vi "Get Selected Controls.vi"(8 "error in (no error)":errorcluster, 10 "List of Properties":string[](array[string]), 11 "Data in":T2) -> (0 "error out":errorcluster, 3 "Selected Ctrls":T1)   [LabVIEW 2020, in "Control Property Tree.lvlib"]
uses:
  Control Property Tree.lvlib
  Module Data--cluster.ctl
  Ctrl Properties Map Data.ctl
  Property array.ctl
  Selected Ctrls - List of Controls.ctl
  Selected Ctrls - List of Properties.ctl
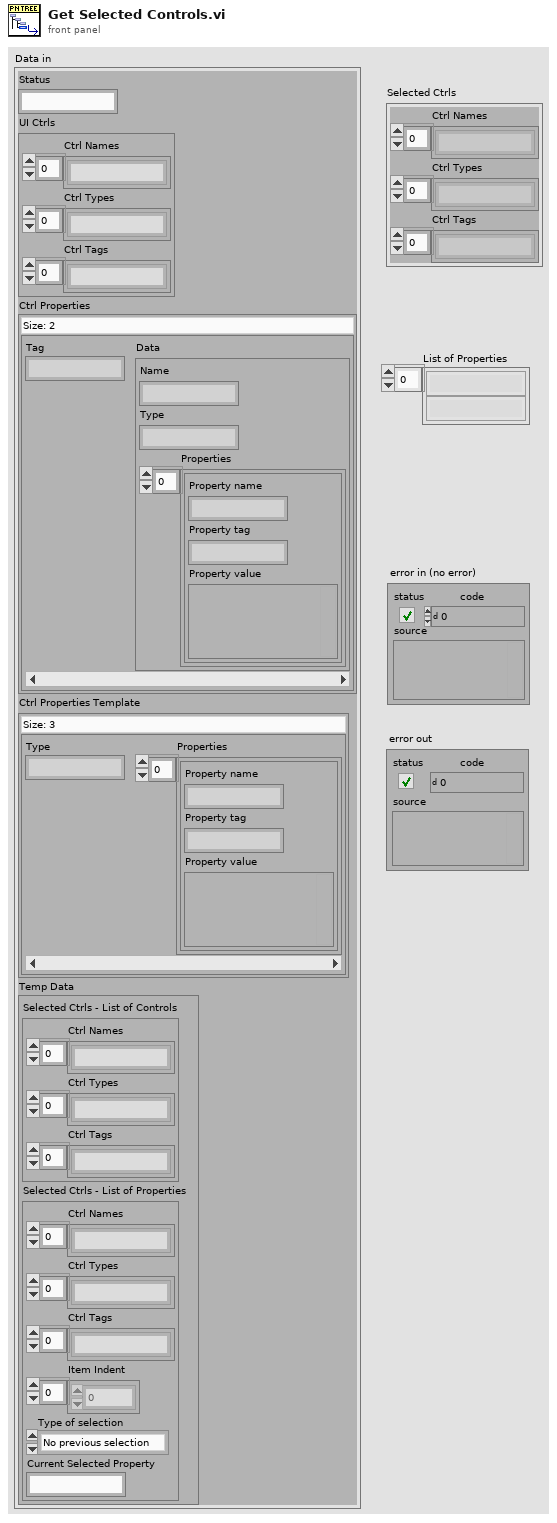
[diagram p1: front panel]
types:
  T1 = cluster{"Ctrl Names":string[], "Ctrl Types":string[], "Ctrl Tags":string[]}
  T2 = typedef "Control Property Tree.lvlib/Module Data--cluster.ctl" = cluster{"Status":string, "UI Ctrls":cluster{"Ctrl Names":string[], "Ctrl Types":string[], "Ctrl Tags":string[]}, "Ctrl Properties":map{string, T3}, "Ctrl Properties Template":map{string, T4}, "Temp Data":cluster{"Selected Ctrls - List of Controls":T5, "Selected Ctrls - List of Properties":T6}}
  T3 = typedef "Control Property Tree.lvlib/Ctrl Properties Map Data.ctl" = cluster{"Name":string, "Type":string, "Properties":T4}
  T4 = typedef "Control Property Tree.lvlib/Property array.ctl" = cluster{"Property name":string, "Property tag":string, "Property value":variant}[]
  T5 = typedef "Control Property Tree.lvlib/Selected Ctrls - List of Controls.ctl" = cluster{"Ctrl Names":string[], "Ctrl Types":string[], "Ctrl Tags":string[]}
  T6 = typedef "Control Property Tree.lvlib/Selected Ctrls - List of Properties.ctl" = cluster{"Ctrl Names":string[], "Ctrl Types":string[], "Ctrl Tags":string[], "Item Indent":i32[], "Type of selection":enum16{"No previous selection", "Control selected", "Property selected"}, "Current Selected Property":string}
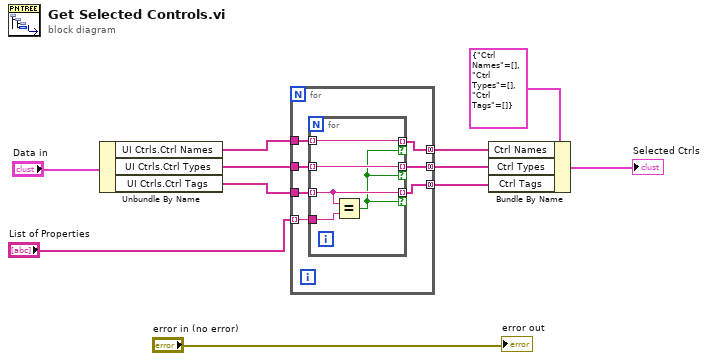
[diagram p0: block diagram]
diagram:
  n1 = Unbundle By Name("Data in") -> ("UI Ctrls.Ctrl Names"=w10:string[], "UI Ctrls.Ctrl Types"=w9:string[], "UI Ctrls.Ctrl Tags"=w8:string[])
  n2 = for {
    tunnel: "List of Properties" -> [w18] mode=indexing
    tunnel: w10 -> [w17]
    tunnel: w9 -> [w16]
    tunnel: w8 -> [w15]
    tunnel: [w14] -> w6 mode=concatenating
    tunnel: [w13] -> w5 mode=concatenating
    tunnel: [w12] -> w4 mode=concatenating
    n3 = for {
      tunnel: w15 -> [w20] mode=indexing
      tunnel: w18 -> [w23]
      tunnel: w17 -> [w22] mode=indexing
      tunnel: w16 -> [w21] mode=indexing
      tunnel: [w22] -> w14 mode=indexing if=w19
      tunnel: [w21] -> w13 mode=indexing if=w19
      tunnel: [w20] -> w12 mode=indexing if=w19
      n4 = Equal?(x=w20, y=w23) -> (x = y?=w19:bool)
    }
  }
  n5 = Bundle By Name(cluster=T1 {"Ctrl Names"=[], "Ctrl Types"=[], "Ctrl Tags"=[]} ("Selected Ctrls"), "Ctrl Names"=w6, "Ctrl Types"=w5, "Ctrl Tags"=w4) -> (→"Selected Ctrls":T1)
  "error out" <- "error in (no error)"
